vi "Remove NAN rows.vi"(6 "Transpose":bool=TRUE, 11 "Array - Numeric":dbl[][](array[numeric])) -> (3 "Array out":dbl[][](array[numeric]))   [LabVIEW 2014]
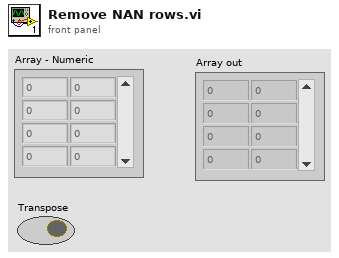
[diagram p1: front panel]
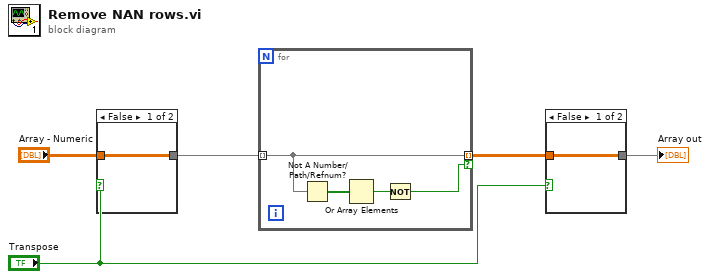
[diagram p0: block diagram]
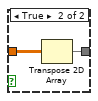
[diagram p2: hidden frame]
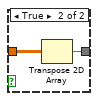
[diagram p3: hidden frame]
diagram:
  n1 = case shown="False" "Transpose" {
    tunnel: "Array - Numeric" -> [w6 w8]
    tunnel: [w6 w7] -> w4
    frame False {
    }
    frame True {
      n2 = Transpose 2D Array(2D array=w8) -> (transposed array=w7:dbl[][])
    }
  }
  n3 = for {
    tunnel: w4 -> [w11] mode=indexing
    tunnel: [w11] -> w2 mode=indexing if=w9
    n4 = Not A Number/Path/Refnum?(number/path/refnum=w11) -> (NaN/Path/Refnum?=w12:bool[])
    n5 = Or Array Elements(Boolean array=w12) -> (logical OR=w10:bool)
    n6 = Not(x=w10) -> (.not. x?=w9:bool)
  }
  n7 = case shown="False" "Transpose" {
    tunnel: w2 -> [w13 w15]
    tunnel: [w13 w14] -> w1
    frame False {
    }
    frame True {
      n8 = Transpose 2D Array(2D array=w15) -> (transposed array=w14:dbl[][])
    }
  }
  "Array out" <- w1
